vi "pp3_log_toString_trialFromStateInfo.vi"(8 "State Info In":T1={"Curr  tr"=0, "Curr (ms)"=0, "Cum (ms)"=0, "Run loop diff"=0, "Tone countdown (ms)"=0, "Countdown (ms)"=0, "Curr State"=enum."0 NULL", "Prev State"=enum."1 Habituation", "Rw"=FALSE, "Sw"=FALSE, "Tone\nGate"=FALSE, "Punish"=FALSE, "Current DAQ DO Int"=0, "Current Loaded Trial"={"Trial Type Number"=1, "Trial Type"=enum."GO", "Trial Weight"=100, "Shock (mA)"=0.3, "Duration (ms)"=0.25, "Sound Type"=enum."04 FM Sweep", "Stim P1"=4000.0, "Stim P2"=0.0, "Stim P3"=0.0, "Stim P4"=2000.0, "DAQ Amplitude (V)"=0.25}, "Total trials memo"=0, "State start cum memo (ms)"=0, "Last dur jump time memo (ms)"=0, "Last dur shock time memo (ms)"=0, "Tone repeat memo (ms)"=0, "Webcam on"=FALSE, "Webcam recording"=FALSE, "State update flag"=FALSE, "Last loaded shock voltage"=0.0, "Vid upd"=enum."0", "First time tone"=FALSE} {"Current DAQ DO Int" format="%016b"; "Current Loaded Trial"."DAQ Amplitude (V)" min=0.0 max=5.0 format="%_4g"; "Current Loaded Trial"."Shock (mA)" min=-1.0 max=5.0; "Current Loaded Trial"."Trial Weight" step=1; "Current Loaded Trial"."Duration (ms)" min=0.0 max=1.0; "Current Loaded Trial"."Trial Type Number" min=1 max=256 step=1}) -> (0 "TRIALMEMO String":string, 3 "spreadsheet string":string)   [LabVIEW 2013]
uses:
  CTL_pp3c_LoopState.ctl
  pp3_CTL_BehavioralState.ctl
  pp3_CTL_Trial.ctl
  pp3_CTL_TrialType.ctl
  labolabo2/waveforms/WFTypes.ctl
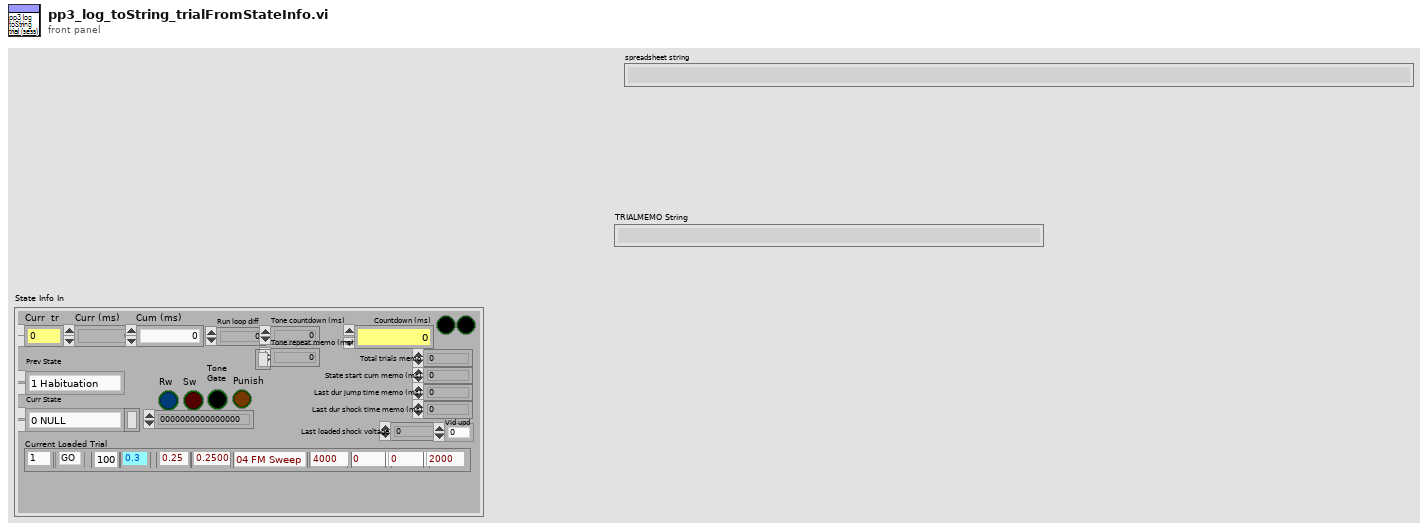
[diagram p1: front panel]
types:
  T1 = typedef "CTL_pp3c_LoopState.ctl" = cluster{"Curr  tr":u16, "Curr (ms)":u32, "Cum (ms)":u64, "Run loop diff":i64, "Tone countdown (ms)":i64, "Countdown (ms)":i64, "Curr State":T2, "Prev State":T2, "Rw":bool, "Sw":bool, "Tone\nGate":bool, "Punish":bool, "Current DAQ DO Int":u16, "Current Loaded Trial":T3, "Total trials memo":i64, "State start cum memo (ms)":i64, "Last dur jump time memo (ms)":i64, "Last dur shock time memo (ms)":i64, "Tone repeat memo (ms)":i64, "Webcam on":bool, "Webcam recording":bool, "State update flag":bool, "Last loaded shock voltage":dbl, "Vid upd":enum16{"0", "1", "2", "3", "4", "5", "6", "7", "8", "9"}, "First time tone":bool}
  T2 = typedef "pp3_CTL_BehavioralState.ctl" = enum8{"0 NULL", "1 Habituation", "2 (Load Trial)", "3 Stay Period", "4 Load Audio/Click Delay", "5 GO Trial", "6 GO Jumped", "7 GO Timeout", "8 NOGO Trial", "9 NOGO Jumped", "10 NOGO Timeout", "11 TEST Trial", "12 TEST Jumped", "13 TEST Timeout", "14 Intertrial Interval", "15 Done"}
  T3 = typedef "pp3_CTL_Trial.ctl" = cluster{"Trial Type Number":i16, "Trial Type":T4, "Trial Weight":u32, "Shock (mA)":dbl, "Duration (ms)":dbl, "Sound Type":T5, "Stim P1":dbl, "Stim P2":dbl, "Stim P3":dbl, "Stim P4":dbl, "DAQ Amplitude (V)":dbl}
  T4 = typedef "pp3_CTL_TrialType.ctl" = enum16{"OFF", "GO", "NOGO", "TEST"}
  T5 = typedef "WFTypes.ctl" = enum16{"00 NULL", "01 DC", "02 Noise", "03 Pure Tone", "04 FM Sweep"}
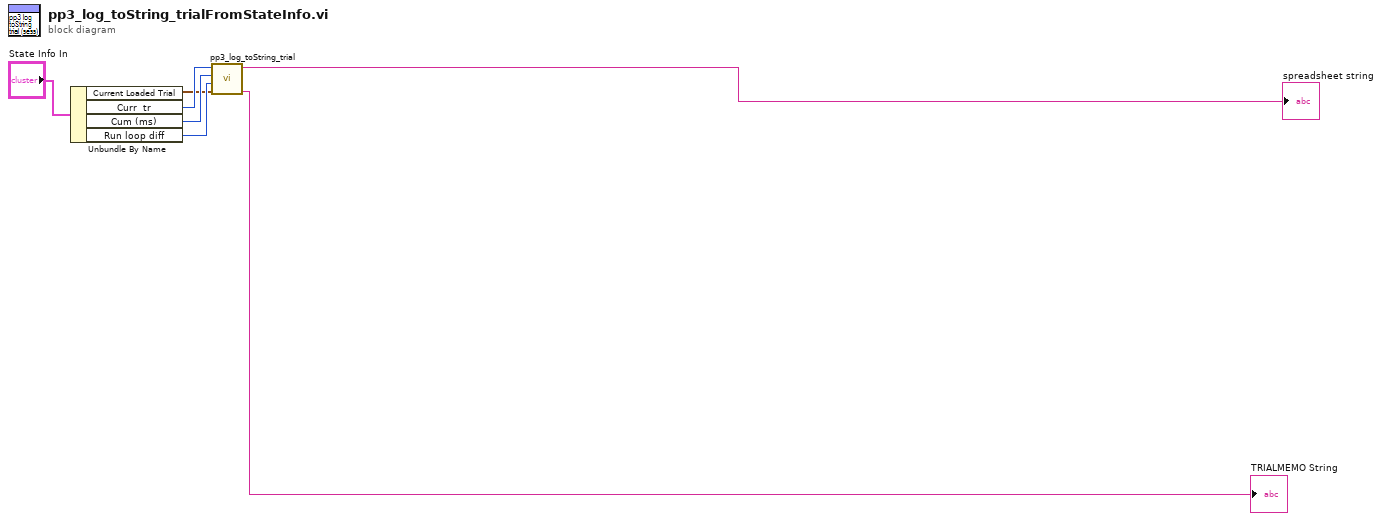
[diagram p0: block diagram]
diagram:
  n1 = Unbundle By Name("State Info In") -> ("Current Loaded Trial"=w1:T3, "Curr  tr"=w4:u16, "Cum (ms)"=w3:u64, "Run loop diff"=w2:i64)
  n2 = call "pp3_log_toString_trial.vi"("input cluster"=w1, "Run loop diff"=w2, "Cum (ms)"=w3, "Curr tr"=w4) -> ("TRIALMEMO String"=→"TRIALMEMO String":string, "spreadsheet string"=→"spreadsheet string":string)  [unwired: 6 in]
